vi "Celsius to Fahrenheit.vi"(10 "Celsius":dbl(slide) scale=0.0..10.0) -> (2 "Fahrenheit":dbl(slide) scale=0.0..100.0)   [LabVIEW 2019]
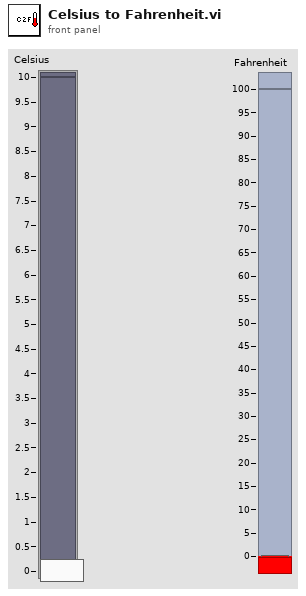
[diagram p1: front panel]
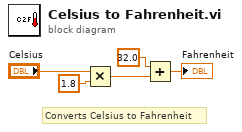
[diagram p0: block diagram]
diagram:
  # "Converts Celsius to Fahrenheit"
  n1 = Multiply(x="Celsius", y=1.8) -> (x*y=w3:dbl)
  n2 = Add(x=32.0, y=w3) -> (x+y=→"Fahrenheit":dbl)
